vi "Run.vi"(11 "Nav6DevRef":T1) -> ()   [LabVIEW 2013, in "Nav6.lvlib"]
doc: "Reads the data from the Nav6 and makes it availible to the Get VIs.\n\nThe Run VI contains an infinite while loop and should be placed in periodic tasks (similar to the compressor run)."
uses:
  Nav6.lvlib
  Nav6DevRef.ctl
  <vilib>/Rock Robotics/WPI/SerialPort/WPI_SerialPortRef.ctl
  Nav6Mode.ctl
  StopGlobal.vi
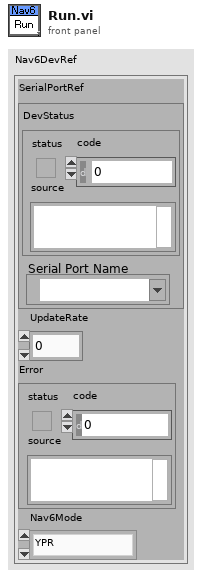
[diagram p1: front panel]
types:
  T1 = typedef "Nav6.lvlib/Nav6DevRef.ctl" = cluster{"SerialPortRef":T2, "UpdateRate":u8, "Error":errorcluster, "Nav6Mode":T3}
  T2 = typedef "WPI_SerialPortRef.ctl" = cluster{"DevStatus":errorcluster, "Serial Port Name":refnum<visa-resource-name>}
  T3 = typedef "Nav6.lvlib/Nav6Mode.ctl" = enum16{"YPR", "Gyro", "Quaternion"}
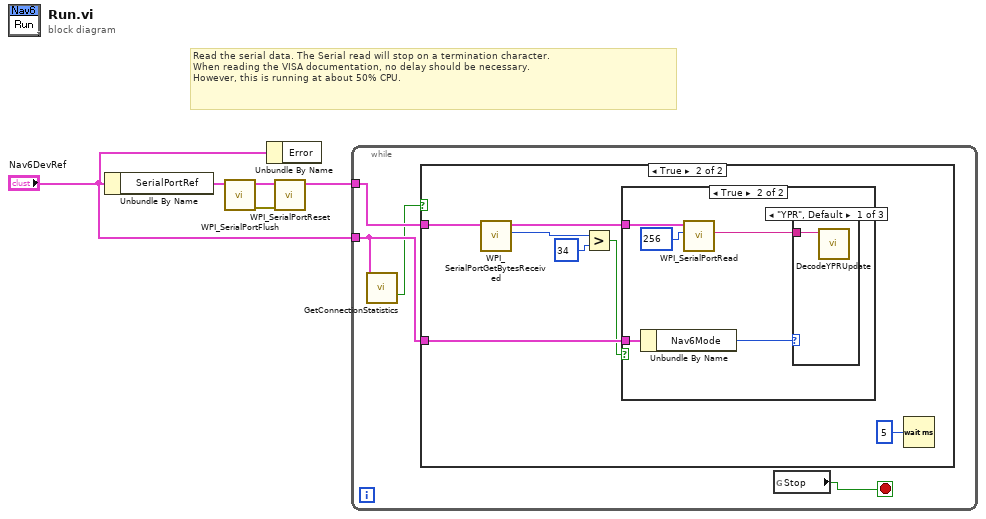
[diagram p0: block diagram]
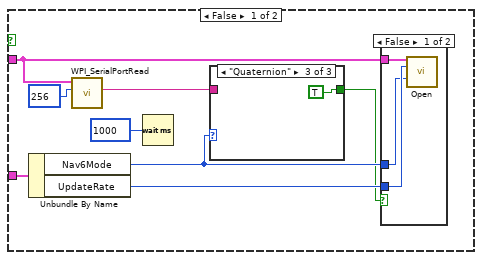
[diagram p2: hidden frame]
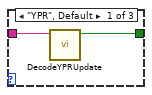
[diagram p4: hidden frame]
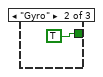
[diagram p5: hidden frame]
diagram:
  # "Read the serial data. The Serial read will stop on a termination character.\nWhen reading the VISA documentation, no delay should be necessary. \nHowever, this is running at about 50% CPU."
  n1 = Unbundle By Name("Nav6DevRef") -> ("SerialPortRef"=w2:T2)
  n2 = call <vilib>:"WPI_SerialPortFlush.vi"("SerialPortRef"=w2) -> ("error out"=w5:errorcluster, "SerialPortRef"=w4:T2)  [unwired: 9 in]
  n3 = Unbundle By Name("Nav6DevRef") -> ()  [unwired: 1 out]
  n4 = call <vilib>:"WPI_SerialPortReset.vi"("error in (no error)"=w5, "SerialPortRef"=w4) -> ("SerialPortRef"=w3:T2)  [unwired: 8 in, 1 out]
  n5 = while {
    tunnel: w3 -> [w9]
    tunnel: "Nav6DevRef" -> [w7]
    stop <- w8 stop-if-true
    n6 = call "GetConnectionStatistics.vi"("Nav6DevRef"=w7) -> ("IsConnected"=w6:bool)  [unwired: 10 in, 4 out]
    n7 = case shown="True" w6 {
      tunnel: w9 -> [w13 w29]
      tunnel: w7 -> [w14 w31]
      frame False {
        n8 = Unbundle By Name(w14) -> ("Nav6Mode"=w11:T3, "UpdateRate"=w12:u8)
        n9 = call <vilib>:"WPI_SerialPortRead.vi"("Num Bytes to Read"=u32 256, "SerialPortRef"=w13) -> ("Buffer"=w16:string)  [unwired: 7 in, 2 out]
        n10 = Wait (ms)(milliseconds to wait=u32 1000) -> ()  [unwired: 1 out]
        n11 = case shown="\"Quaternion\"" w11 {
          tunnel: w16 -> [w22 _ _]
          tunnel: [w21 TRUE ("MessageReceived") TRUE ("MessageReceived")] -> w10
          frame "YPR", Default {
            n12 = call "DecodeYPRUpdate.vi"("Buffer"=w22) -> ("MessageReceived"=w21:bool)  [unwired: 10 in]
          }
          frame "Gyro" {
          }
          frame "Quaternion" {
          }
        }
        n13 = case shown="False" w10 {
          tunnel: w13 -> [w20 _]
          tunnel: w12 -> [w19 _]
          tunnel: w11 -> [w18 _]
          frame False {
            n14 = call "Open.vi"("SerialPortRef"=w20, "UpdateRate (100Hz)"=w19, "Nav6Mode (YPR)"=w18) -> ()  [unwired: 6 in, 7 out]
          }
          frame True {
          }
        }
      }
      frame True {
        n15 = call <vilib>:"WPI_SerialPortGetBytesReceived.vi"("SerialPortRef"=w29) -> ("Bytes at Port"=w27:u32, "SerialPortRef"=w28:T2)  [unwired: 8 in, 1 out]
        n16 = Greater?(x=w27, y=u32 34) -> (0:w25:bool)
        n17 = case shown="True" w25 {
          tunnel: w31 -> [_ w35]
          tunnel: w28 -> [_ w33]
          frame False {
          }
          frame True {
            n18 = Unbundle By Name(w35) -> ("Nav6Mode"=w34:T3)
            n19 = call <vilib>:"WPI_SerialPortRead.vi"("Num Bytes to Read"=u32 256, "SerialPortRef"=w33) -> ("Buffer"=w36:string)  [unwired: 7 in, 2 out]
            n20 = case shown="\"YPR\", Default" w34 {
              tunnel: w36 -> [w37 _ _]
              frame "YPR", Default {
                n21 = call "DecodeYPRUpdate.vi"("Buffer"=w37) -> ()  [unwired: 10 in, 1 out]
              }
              frame "Gyro" {
              }
              frame "Quaternion" {
              }
            }
          }
        }
        n22 = Wait (ms)(milliseconds to wait=u32 5) -> ()  [unwired: 1 out]
      }
    }
    n23 = global read "StopGlobal.vi" "Stop"() -> (w8:bool)
  }
